vi "Write_Data.vi"(8 "error in (no error)":errorcluster caption="entrée d'erreur (pas d'erreur)", 10 "Data_To_Write":string, 11 "Class DIO en entrée":refnum<class "Class Instrument DIO.lvclass">) -> (0 "error out":errorcluster caption="sortie d'erreur", 3 "Class DIO en Sortie":refnum<class "Class Instrument DIO.lvclass">)   [LabVIEW 2020, in "Library Instrument & Equipement.lvlib" / "Library Instruments.lvlib" / "Class Instrument DIO.lvclass"]
uses:
  Class Instrument DIO.lvclass
  JSON API/JSON Value/Set from JSON string.vi
  JSON API/JSON Value/JSON Value.lvclass
  Class Instrument DIO.lvclass/Class Instrument DIO.ctl
  JSON API/Variant JSON/Variant JSON.lvlib
  JSON API/Get Polymorphic/JSON GetSet.lvlib
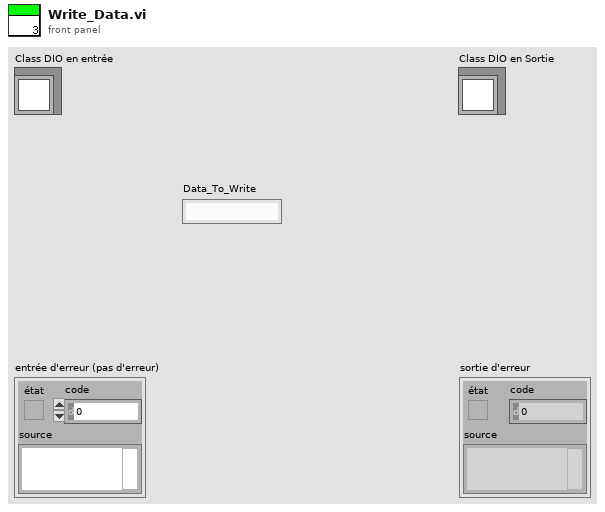
[diagram p1: front panel]
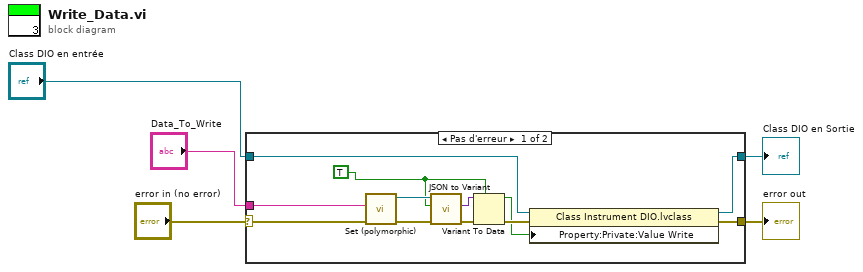
[diagram p0: block diagram]
diagram:
  n1 = case shown="Pas d'erreur" "error in (no error)" {
    selector: "error in (no error)" -> [w9 w19]
    tunnel: [w16 w19] -> w4
    tunnel: [w15 w18] -> w2
    tunnel: "Class DIO en entrée" -> [w17 w18]
    tunnel: "Data_To_Write" -> [w10 _]
    frame No Error {
      w7 = TRUE
      n2 = call-poly "Set (polymorphic).vi"("error in (no error)"=w9, "JSON stream"=w10) -> ("error out"=w13:errorcluster, "JSON Value out"=w11:refnum<class "JSON Value.lvclass">)  [unwired: 7 in, 1 out]
      n3 = call "JSON to Variant.vi"("error in (no error)"=w13, "Variant (Data Type)"=w7, "JSON Value"=w11) -> ("error out"=w12:errorcluster, "Variant out"=w14:variant)  [unwired: 7 in]
      n4 = Variant To Data(error in=w12, type=w7, Variant=w14) -> (data=w6:bool, error out=w8:errorcluster)
      n5 = property class="Class Instrument DIO.lvclass"(reference=w17, error in=w8, "Property:Private:Value Write"=w6) -> (reference out=w15:refnum<class "Class Instrument DIO.lvclass">, error out=w16:errorcluster)
    }
    frame Error {
    }
  }
  "error out" <- w4
  "Class DIO en Sortie" <- w2
